vi "Hardware整体图.vi"() -> ()   [LabVIEW 2014]
panel:
  in  "Pda":bool
  in  "Pcmcia":bool
  in  "Pci":bool
  in  "Mouse":bool
  in  "Modem":bool
  in  "Memory":bool
  in  "Info":bool
  in  "Hdd":bool
  in  "Flash":bool
  in  "Flash disk":bool
  in  "Dat":bool
  in  "Cpu":bool
  in  "Control":bool
  in  "Battery":bool
  in  "Zip drive":bool
  in  "Usb":bool
  in  "Tablet":bool
  in  "Simulation":bool
  in  "Sharing":bool
  in  "Settings":bool
  in  "Set":bool
  in  "Scanner":bool
  in  "Scan":bool
  in  "Router":bool
  in  "Raid":bool
  in  "Processor":bool
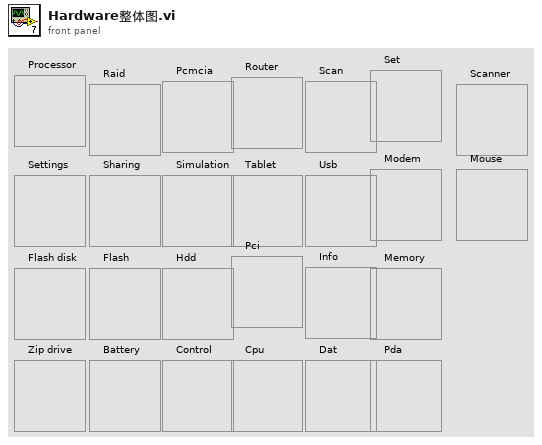
[diagram p1: front panel]
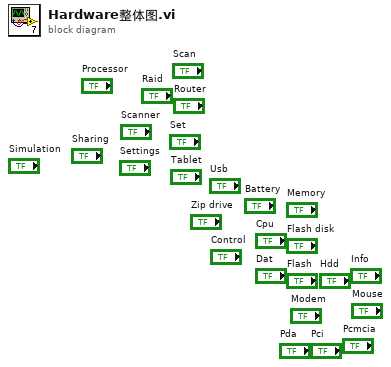
[diagram p0: block diagram]
diagram:
